vi "laserGetTemp.vi"(8 "error in (no error)":errorcluster, 9 "tmax (C, default = 38)":dbl=35.0, 10 "milliseconds to wait":u32=5, 11 "VISA resource name":refnum<visa-resource-name>) -> (0 "error out":errorcluster, 1 "Overtemp":bool, 2 "Temp (C)":dbl, 3 "VISA resource name out":refnum<visa-resource-name>)   [LabVIEW 2011]
panel:
  out "return byte count":u32
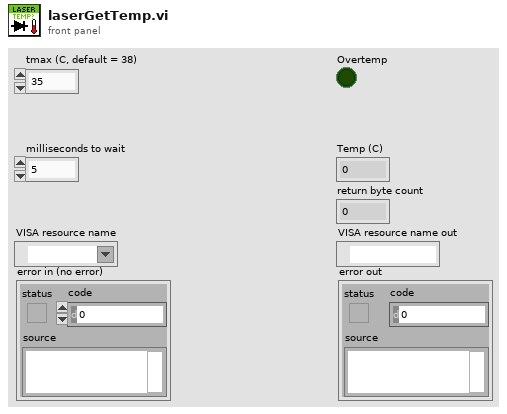
[diagram p1: front panel]
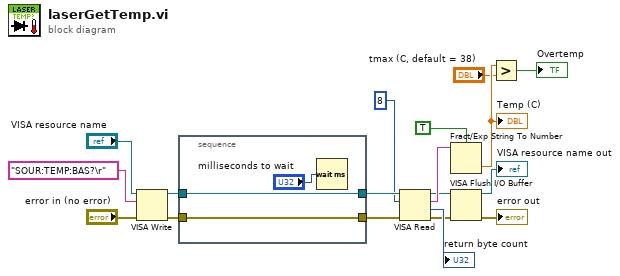
[diagram p0: block diagram]
diagram:
  n1 = VISA Write(VISA resource name="VISA resource name", write buffer="SOUR:TEMP:BAS?\r", error in (no error)="error in (no error)") -> (VISA resource name out=w17:refnum<visa-resource-name>, error out=w16:errorcluster)  [unwired: 1 out]
  n2 = stacked-sequence {
    tunnel: w17 -> [w21]
    tunnel: [w21] -> w15
    tunnel: [w20] -> w14
    tunnel: w16 -> [w20]
    frame #0 {
      n3 = Wait (ms)(milliseconds to wait="milliseconds to wait") -> ()  [unwired: 1 out]
    }
  }
  n4 = VISA Read(VISA resource name=w15, byte count=u32 8, error in (no error)=w14) -> (VISA resource name out=w7:refnum<visa-resource-name>, read buffer=w12:string, return count=→"return byte count":u32, error out=w6:errorcluster)
  n5 = Fract/Exp String To Number(use system decimal point (T)=TRUE, string=w12) -> (number=w3:dbl)  [unwired: 2 in, 1 out]
  "Temp (C)" <- w3
  n6 = VISA Flush I/O Buffer(VISA resource name=w7, error in (no error)=w6) -> (VISA resource name out=→"VISA resource name out":refnum<visa-resource-name>, error out=→"error out":errorcluster)  [unwired: 1 in]
  n7 = Greater?(x=w3, y="tmax (C, default = 38)") -> (0:→"Overtemp":bool)
